vi "GLdrv_MEAS_TIME.vi"(0 "Connection ID":T1, 11 "error in (no error)":errorcluster) -> (4 "Connection ID Out":T1, 6 "Start Time":string, 8 "Stop Time":string, 10 "Trigger Time":string, 15 "error out":errorcluster)   [LabVIEW 2017, in "GL860_Driver.lvlib"]
doc: "測定開始時刻,測定終了時刻,トリガ時刻を参照します"
uses:
  GL860_Driver.lvlib
  ConnectionID.ctl
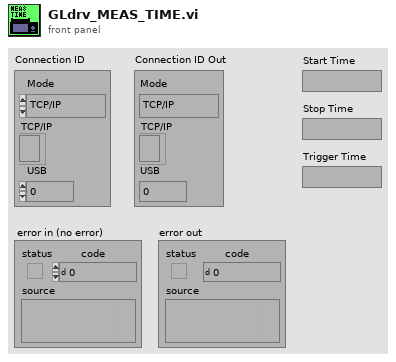
[diagram p1: front panel]
types:
  T1 = typedef "ConnectionID.ctl" = cluster{"Mode":enum16{"TCP/IP", "USB"}, "TCP/IP":refnum<k5>, "USB":i32}
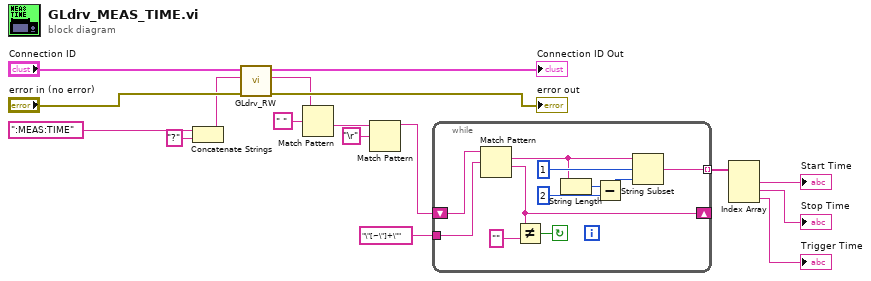
[diagram p0: block diagram]
diagram:
  n1 = Concatenate Strings(":MEAS:TIME" ("Command"), "?" ("string")) -> (w8:string)
  n2 = call "GLdrv_RW.vi"("error in (no error)"="error in (no error)", "data in"=w8, "Connection ID"="Connection ID") -> ("error out"=→"error out":errorcluster, "data out"=w7:string, "Connection ID Out"=→"Connection ID Out":T1)  [unwired: 4 in, 2 out]
  n3 = Match Pattern(string=w7, regular expression=" " ("search string/char (-)")) -> (after substring=w10:string)  [unwired: 4 out]
  n4 = Match Pattern(string=w10, regular expression="\r") -> (before substring=w5:string)  [unwired: 4 out]
  n5 = while {
    tunnel: [w19] -> w4 mode=indexing
    shift-right: [w27] -> _
    shift-left: w5 -> [w28]
    tunnel: "\"[~\"]+\"" ("regular expression") -> [w18]
    stop <- w25 continue-if-true
    n6 = Match Pattern(string=w28, regular expression=w18) -> (match substring=w20:string, after substring=w27:string)  [unwired: 3 out]
    n7 = Not Equal?(x=w27, y="") -> (x != y?=w25:bool)
    n8 = String Length(string=w20) -> (length=w22:i32)
    n9 = Subtract(x=w22, y=2) -> (x-y=w23:i32)
    n10 = String Subset(string=w20, offset (0)=1, length (rest)=w23) -> (substring=w19:string)
  }
  n11 = Index Array(array=w4) -> (element #1=→"Start Time":string, element #2=→"Stop Time":string, element #3=→"Trigger Time":string)  [unwired: 3 in]
